vi "Prueba.vi"() -> ()   [LabVIEW 2014, in "AD4212C Lib.lvlib"]
uses:
  AD4212C Lib.lvlib
  Typedef/Connection Data.ctl
panel:
  out "Value":dbl format="%.2f"
  out "VISA resource name Out":T1={"Conection Data"="COM4"}
  out "error out":errorcluster
  in  "VISA resource name In":T1={"Conection Data"="COM4"}
  in  "error in (no error)":errorcluster
  in  "Read":bool
  in  "Configuration":bool
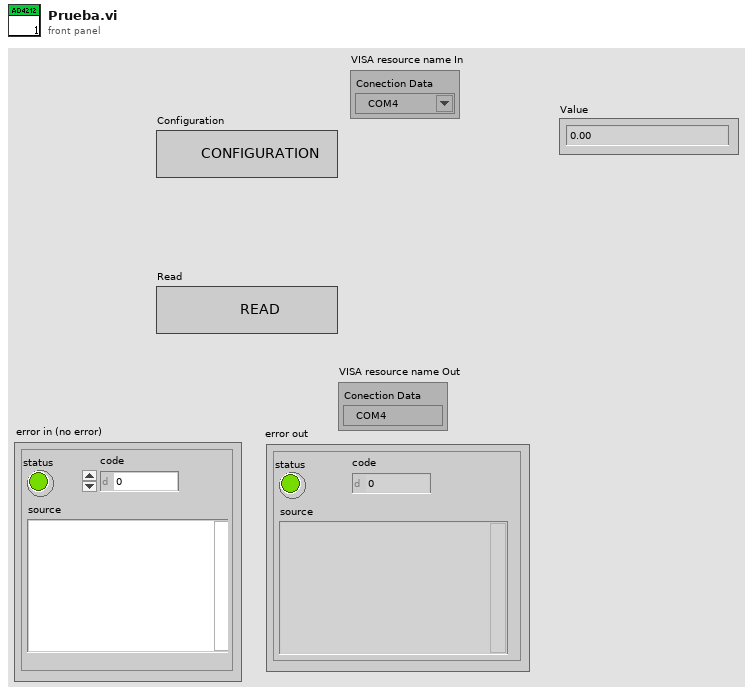
[diagram p1: front panel]
types:
  T1 = typedef "AD4212C Lib.lvlib/Connection Data.ctl" = cluster{"Conection Data":refnum<visa-resource-name>}
  T2 = enum16{"Idle Init", "Init", "Read", "AutoRefresh", "Stop", "Close", "Idle Close"}
  T3 = enum16{"Init", "Idle Init", "Star", "Read", "AutoRefresh", "Stop", "Close", "Idle Close"}
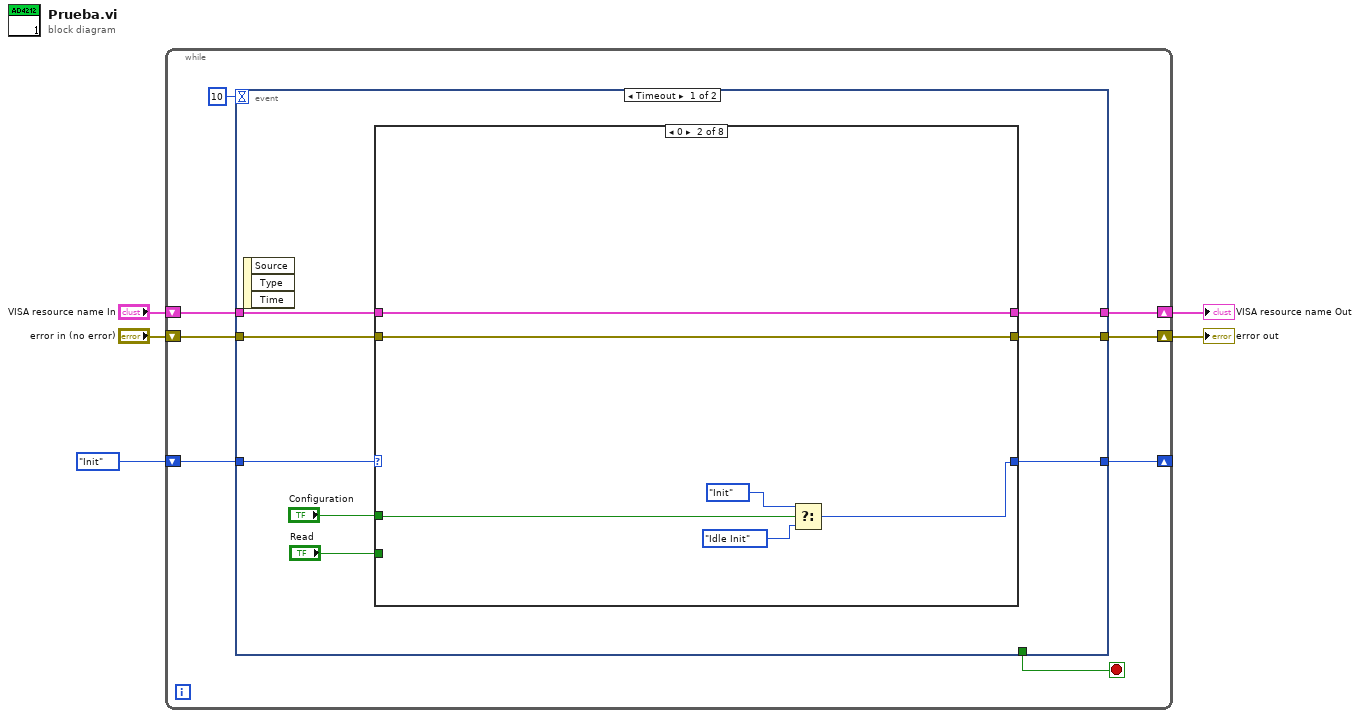
[diagram p0: block diagram]
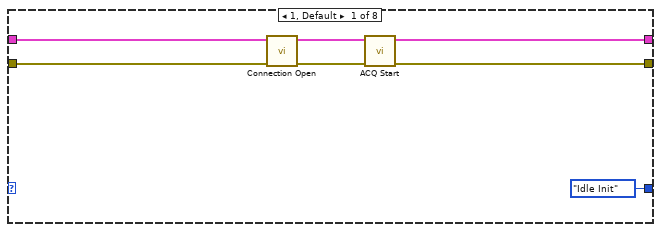
[diagram p2: hidden frame]
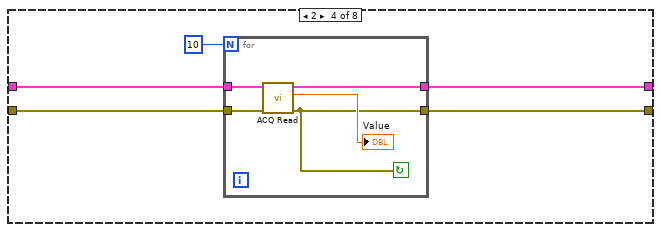
[diagram p4: hidden frame]
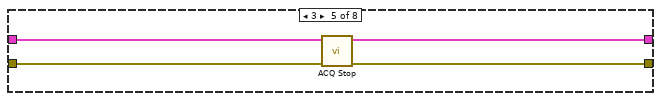
[diagram p5: hidden frame]
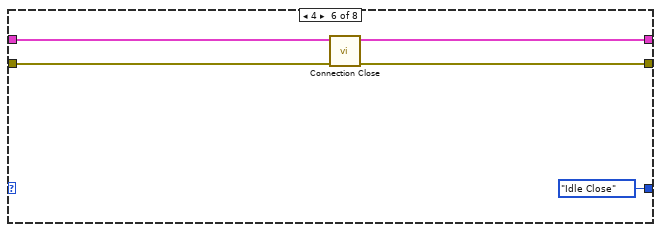
[diagram p6: hidden frame]
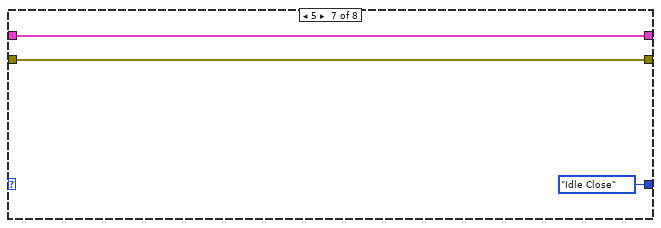
[diagram p7: hidden frame]
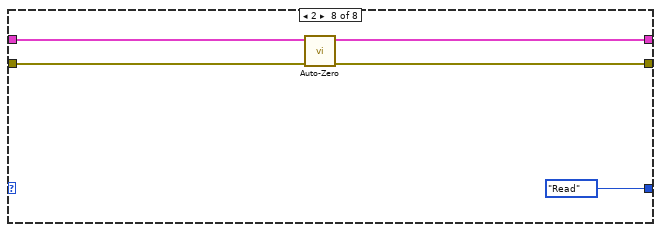
[diagram p8: hidden frame]
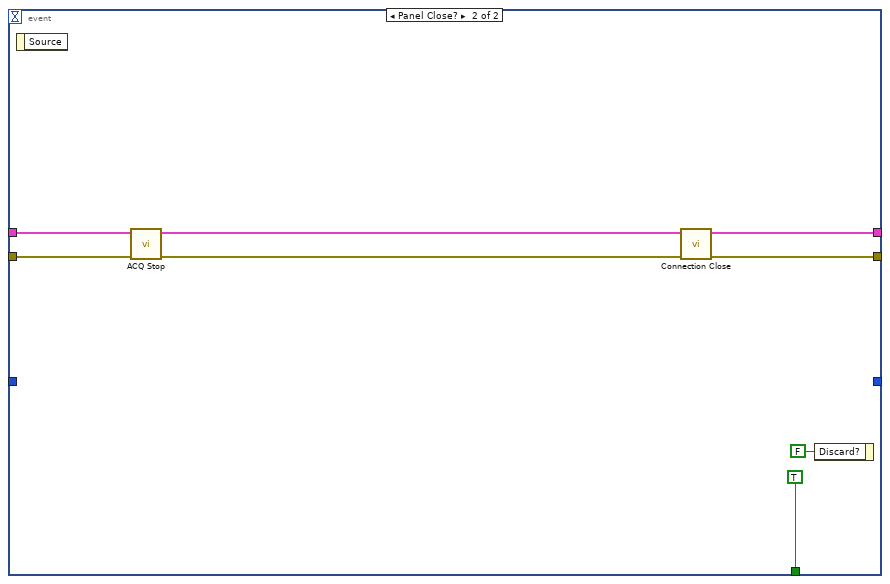
[diagram p9: hidden frame]
diagram:
  n1 = while {
    shift-right: [w11] -> w4
    shift-left: "VISA resource name In" -> [w12]
    shift-right: [w10] -> w3
    shift-left: "error in (no error)" -> [w9]
    shift-right: [w6] -> _
    shift-left: T2."Init" -> [w7]
    stop <- w13 stop-if-true
    n2 = event shown="[0] Timeout" {
      selector: _ -> [_ _]
      dyn-events: _ -> [_ _]
      timeout: 10 -> [_ _]
      tunnel: [_ TRUE ("Stop")] -> w13
      tunnel: w12 -> [w21 w63]
      tunnel: [w20 w67] -> w11
      tunnel: [w19 w66] -> w10
      tunnel: w9 -> [w18 w62]
      tunnel: [w17 _] -> w6
      tunnel: w7 -> [w14 _]
      event Timeout {
        n3 = event-data() -> ()  [unwired: 1 in, 3 out]
        n4 = case shown="0" w14 {
          tunnel: w21 -> [w23 w34 _ w38 w48 w53 w55 w61]
          tunnel: [w25 w34 _ w36 w47 w51 w55 w59] -> w20
          tunnel: [w24 w33 _ w35 w46 w50 w54 w58] -> w19
          tunnel: w18 -> [w22 w33 _ w37 w45 w52 w54 w60]
          tunnel: [T3."Idle Init" w30 _ _ _ T3."Idle Close" T3."Idle Close" T3."Read"] -> w17
          tunnel: "Configuration" -> [_ w32 _ _ _ _ _ _]
          tunnel: "Read" -> [_ _ _ _ _ _ _ _]
          frame 1, Default {
            n5 = call "Connection Open.vi"("VISA resource name Out 3"=w23, "error in (no error)"=w22) -> ("VISA resource name Out 2"=w27:T1, "error out"=w26:errorcluster)  [unwired: 7 in]
            n6 = call "ACQ Start.vi"("error in (no error)"=w26, "VISA resource name In"=w27) -> ("error out"=w24:errorcluster, "VISA resource name Out"=w25:T1)  [unwired: 8 in]
          }
          frame 0 {
            n7 = Select(t=T3."Init", s=w32, f=T3."Idle Init") -> (s? t:f=w30:T3)
          }
          frame 2 {
          }
          frame 2 {
            n8 = for {
              N: 10 -> [_]
              tunnel: w37 -> [w42]
              tunnel: [w40] -> w35
              tunnel: w38 -> [w44]
              tunnel: [w43] -> w36
              stop <- w40 continue-if-true
              n9 = call "ACQ Read.vi"("error in (no error)"=w42, "VISA resource name In"=w44) -> ("error out"=w40:errorcluster, "Value"=→"Value":sgl, "VISA resource name Out"=w43:T1)  [unwired: 7 in]
            }
          }
          frame 3 {
            n10 = call "ACQ Stop.vi"("error in (no error)"=w45, "VISA resource name In"=w48) -> ("error out"=w46:errorcluster, "VISA resource name Out"=w47:T1)  [unwired: 8 in]
          }
          frame 4 {
            n11 = call "Connection Close.vi"("error in (no error)"=w52, "VISA resource name In"=w53) -> ("error out"=w50:errorcluster, "VISA resource name Out"=w51:T1)  [unwired: 8 in]
          }
          frame 5 {
          }
          frame 2 {
            n12 = call "Auto-Zero.vi"("error in (no error)"=w60, "VISA resource name In"=w61) -> ("error out"=w58:errorcluster, "VISA resource name Out"=w59:T1)  [unwired: 8 in]
          }
        }
      }
      event Panel Close? {
        n13 = event-data() -> ()  [unwired: 1 in, 1 out]
        n14 = call "ACQ Stop.vi"("error in (no error)"=w62, "VISA resource name In"=w63) -> ("error out"=w64:errorcluster, "VISA resource name Out"=w65:T1)  [unwired: 8 in]
        n15 = call "Connection Close.vi"("error in (no error)"=w64, "VISA resource name In"=w65) -> ("error out"=w66:errorcluster, "VISA resource name Out"=w67:T1)  [unwired: 8 in]
        n16 = event-data("Discard?"=FALSE) -> ()  [unwired: 1 in, 1 out]
      }
    }
  }
  "error out" <- w3
  "VISA resource name Out" <- w4
